vi "Test_test.vi"() -> ()   [LabVIEW 2013]
uses:
  classes/Devices/DeviceInterface/Devices.ctl
  classes/Tests/TestInterface/Tests.ctl
panel:
  in  "Boolesch":bool
  out "Kommentar":string
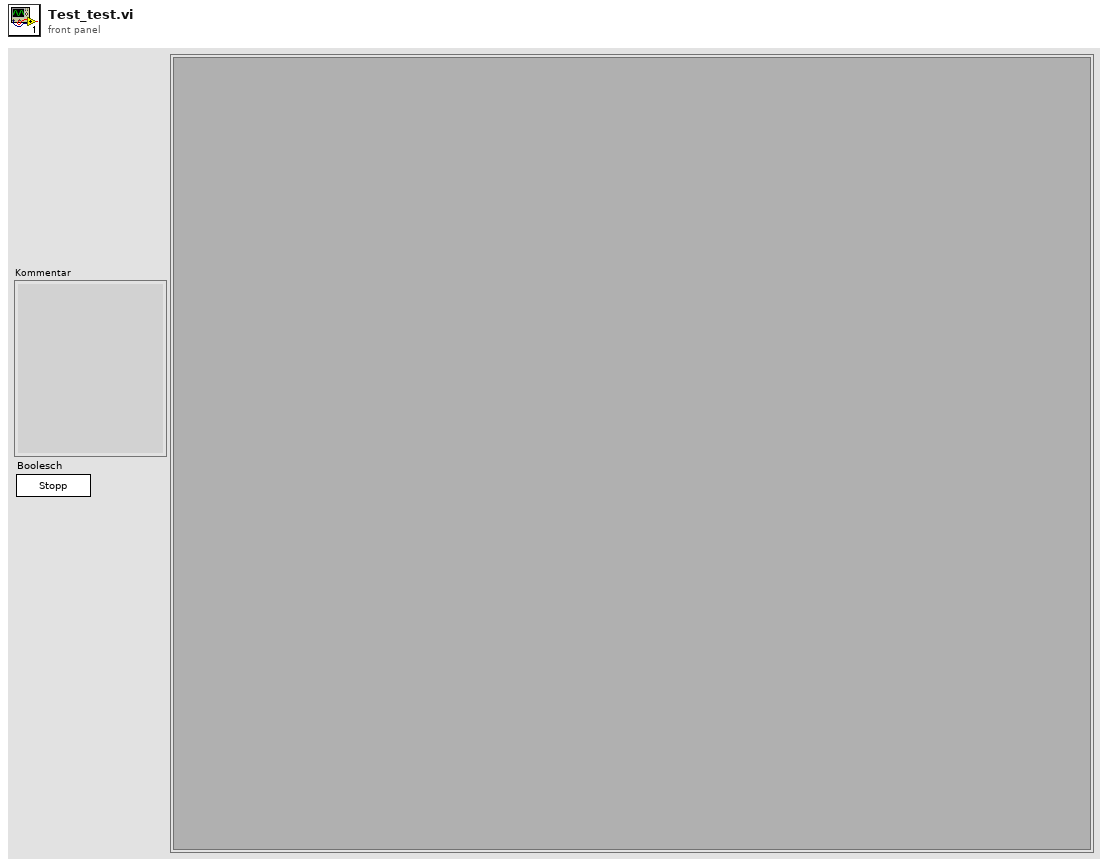
[diagram p1: front panel]
types:
  T1 = typedef "Tests.ctl" = enum16{"Störaussendung", "Burst", "ESD", "Surge", "Spannungseinbruch", "HF-Felder"}
  T2 = typedef "Devices.ctl" = enum16{"Tektronix RSA5106A", "emTestCWS500N", "CEG450"}
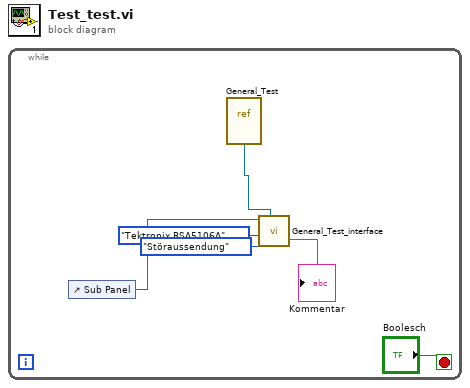
[diagram p0: block diagram]
diagram:
  n1 = while {
    stop <- "Boolesch" stop-if-true
    n2 = control-ref of="Sub Panel"() -> (w6:refnum<vi>)
    n3 = vi-ref "General_Test.vi"() -> (w3:refnum<vi>)
    n4 = call "General_Test_interface.vi"("VI Refnum"=w3, "device"=Devices."Tektronix RSA5106A", "test"=Tests."Störaussendung", "SubPanel in"=w6) -> ("Kommentar"=→"Kommentar":string)  [unwired: 3 in, 4 out]
  }
